vi "Save Coverage Report.vi"(8 "error in (no error)":errorcluster, 10 "Coverage":refnum<class "Coverage.lvclass">, 11 "Path":path) -> (0 "error out":errorcluster)   [LabVIEW 2017, in "Cobertura.lvlib"]
uses:
  Cobertura.lvlib
  Coverage/Coverage.lvclass
  <vilib>/xml/Close Reference(Node).vi
  <vilib>/xml/NI_XML.lvlib
  <resource>/objmgr/DOMUserDefRef.rc
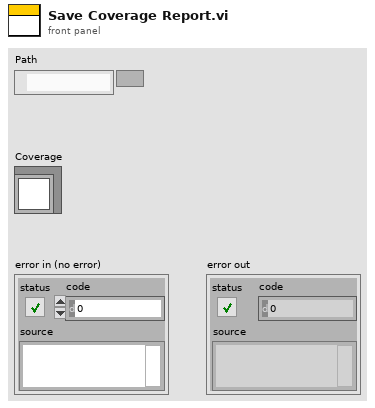
[diagram p1: front panel]
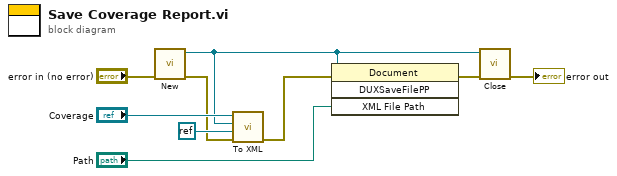
[diagram p0: block diagram]
diagram:
  n1 = call <vilib>:"New.vi"("error in (no error)"="error in (no error)") -> ("error out"=w6:errorcluster, "DOM document out"=w1:refnum<k20>)  [unwired: 7 in]
  n2 = call-dynamic "To XML.vi"("error in (no error)"=w6, "Parent"=refnum<k0> refnum, "Document"=w1, "Coverage in"="Coverage") -> ("error out"=w2:errorcluster)  [unwired: 7 in]
  n3 = invoke class="Document" method="DUXSaveFilePP"(reference=w1, error in=w2, "XML File Path"="Path") -> (error out=w4:errorcluster)  [unwired: 1 in, 3 out]
  n4 = call-poly <vilib>:"Close.vi"("error in (no error)"=w4, "node"=w1) -> ("error out"=→"error out":errorcluster)  [unwired: 7 in]
